vi "Configure Math FFT Function.vi"(6 "FFT Window (0: Rectangular)":i32(ring) items=["Rectangular", "Hanning", "Flattop", "Blackman-Harris", "Hamming"], 7 "Reference Point (0: Display)":i32(ring) items=["Display", "Trigger"], 8 "error in (no error)":errorcluster, 9 "Center Frequency (5E+9 Hz)":dbl=5000000000.0, 10 "Math Channel (1: Function 1)":i32(ring)=1 items=["Function 1"=1, "Function 2"=2, "Function 3"=3, "Function 4"=4, "Function 5"=5, "Function 6"=6, "Function 7"=7, "Function 8"=8, "Function 9"=9, "Function 10"=10, "Function 11"=11, "Function 12"=12, "Function 13"=13, "Function 14"=14, "Function 15"=15, "Function 16"=16], 11 "VISA resource name":refnum<visa-resource-name>) -> (0 "error out":errorcluster, 3 "VISA resource name out":refnum<visa-resource-name>)   [LabVIEW 2020, in "Agilent 90000 Series.lvlib"]
doc: "Configures Fast Fourier Transform function for math operation."
uses:
  Agilent 90000 Series.lvlib
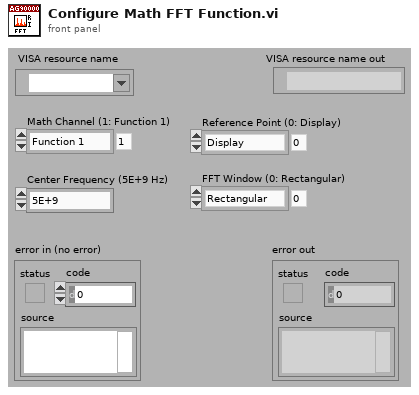
[diagram p1: front panel]
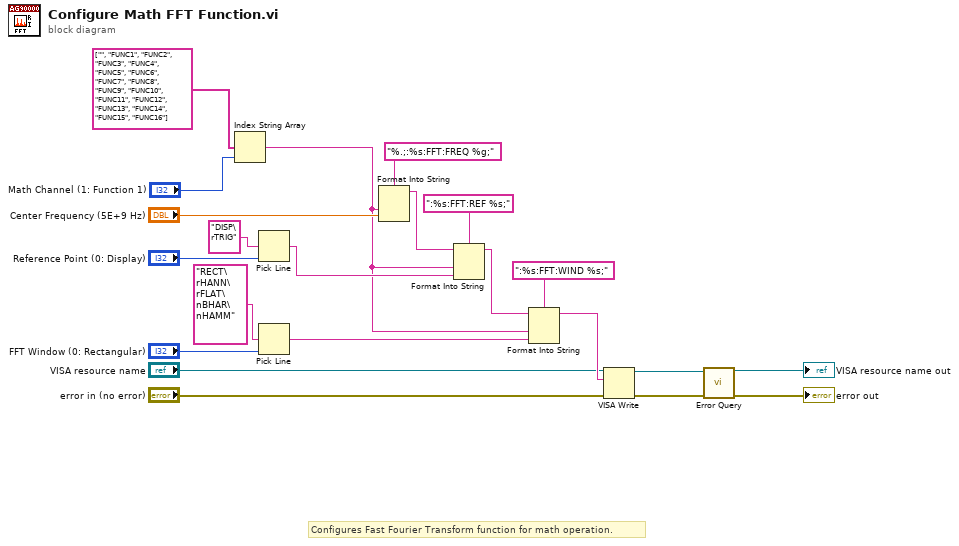
[diagram p0: block diagram]
diagram:
  # "Configures Fast Fourier Transform function for math operation."
  n1 = Index String Array(1:"Math Channel (1: Function 1)", 2:string[] ["", "FUNC1", "FUNC2", "FUNC3", "FUNC4", "FUNC5", "FUNC6", "FUNC7", "FUNC8", "FUNC9", "FUNC10", "FUNC11", "FUNC12", "FUNC13", "FUNC14", "FUNC15", "FUNC16"] ("subarray 2")) -> (0:w2:string)  [unwired: 1 in]
  n2 = Pick Line(multi-line string="DISP\rTRIG", line index="Reference Point (0: Display)") -> (output string=w17:string)  [unwired: 1 out]
  n3 = Pick Line(multi-line string="RECT\rHANN\rFLAT\nBHAR\nHAMM", line index="FFT Window (0: Rectangular)") -> (output string=w12:string)  [unwired: 1 out]
  n4 = Format Into String(format string="%.;:%s:FFT:FREQ %g;", w2, "Center Frequency (5E+9 Hz)") -> (resulting string=w18:string)  [unwired: 2 in, 1 out]
  n5 = Format Into String(format string=":%s:FFT:REF %s;", initial string=w18, w2, w17) -> (resulting string=w13:string)  [unwired: 1 in, 1 out]
  n6 = Format Into String(format string=":%s:FFT:WIND %s;", initial string=w13, w2, w12) -> (resulting string=w11:string)  [unwired: 1 in, 1 out]
  n7 = VISA Write(VISA resource name="VISA resource name", write buffer=w11, error in (no error)="error in (no error)") -> (VISA resource name out=w8:refnum<visa-resource-name>, error out=w7:errorcluster)  [unwired: 1 out]
  n8 = call "Error Query.vi"("error in (no error)"=w7, "VISA resource name"=w8) -> ("error out"=→"error out":errorcluster, "VISA resource name out"=→"VISA resource name out":refnum<visa-resource-name>)  [unwired: 8 out]
